vi "PhotonCount.vi"(9 "# Photons":dbl, 10 "Data in":dbl[](array[numeric]), 11 "Boolean":bool) -> (2 "time out":dbl[](array[numeric]) format="%.2f")   [LabVIEW 2015]
panel:
  in  "Aux":dbl
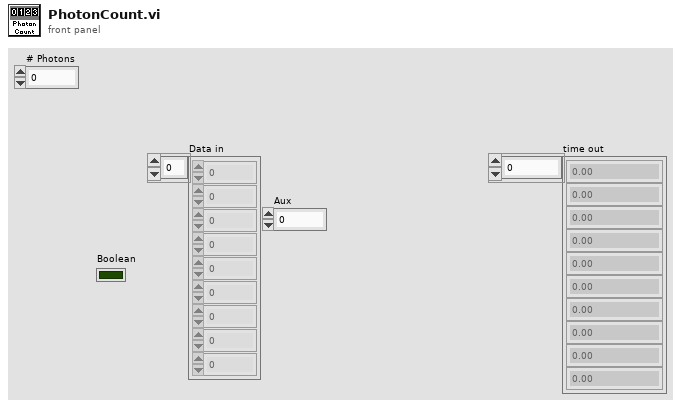
[diagram p1: front panel]
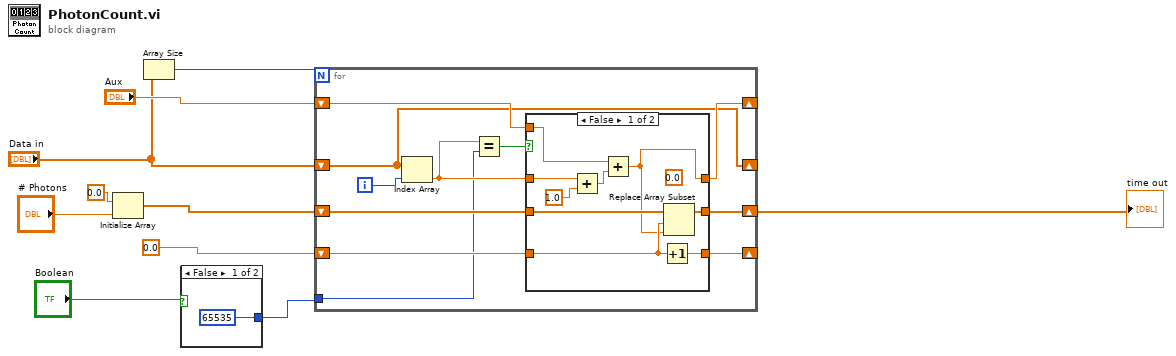
[diagram p0: block diagram]
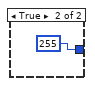
[diagram p2: hidden frame]
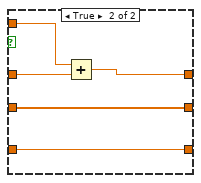
[diagram p3: hidden frame]
diagram:
  n1 = Initialize Array(0.0, "# Photons") -> (w7:dbl[])
  n2 = Array Size(array="Data in") -> (size(s)=w8:i32)
  n3 = case shown="False" "Boolean" {
    tunnel: [u16 65535 ("y") u8 255 ("y")] -> w1
    frame False {
    }
    frame True {
    }
  }
  n4 = for {
    N: w8 -> [_]
    shift-right: [w16] -> _
    shift-left: "Data in" -> [w16]
    shift-right: [w20] -> w9
    shift-left: w7 -> [w21]
    shift-right: [w17] -> _
    shift-left: "Aux" -> [w18]
    shift-right: [w14] -> _
    shift-left: 0.0 ("element") -> [w15]
    tunnel: w1 -> [w13]
    i -> [w23]
    n5 = Index Array(array=w16, index=w23) -> (element=w19:dbl)
    n6 = Equal?(x=w19, y=w13) -> (x = y?=w22:bool)
    n7 = case shown="False" w22 {
      tunnel: w21 -> [w31 w37]
      tunnel: [w30 w37] -> w20
      tunnel: w19 -> [w27 w34]
      tunnel: w18 -> [w28 w35]
      tunnel: [w24 w33] -> w17
      tunnel: w15 -> [w26 w36]
      tunnel: [w25 w36] -> w14
      frame False {
        (unwired) 0.0 ("y")
        n8 = Add(x=w27, y=1.0) -> (x+y=w29:dbl)
        n9 = Add(x=w28, y=w29) -> (x+y=w24:dbl)
        n10 = Increment(x=w26) -> (x+1=w25:dbl)
        n11 = Replace Array Subset(array=w31, new element=w24, index=w26) -> (w30:dbl[])
      }
      frame True {
        n12 = Add(x=w35, y=w34) -> (x+y=w33:dbl)
      }
    }
  }
  "time out" <- w9
